vi "Write Message.vi"(10 "CANopen Message":refnum<class "CANopen Message.lvclass">, 11 "ICAN":refnum<class "ICAN.lvclass">) -> ()   [LabVIEW 2024, in "CANopen Master.lvlib"]
uses:
  CANopen Master.lvlib
  HAL/HAL/Protocols/ICAN/ICAN.lvclass
  CANopen Message/CANopen Message.lvclass
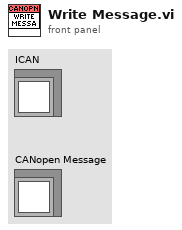
[diagram p1: front panel]
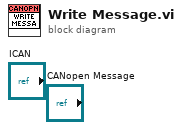
[diagram p0: block diagram]
diagram:
